vi "raster-scanning_sin_est.vi"() -> ()   [LabVIEW 2017]
uses:
  controls/boolean_info.ctl
  raster-scan-params.ctl
  controls/PI-params.ctl
  fpga_subVIs_ssxy/typeDefs/FXP_ss_control_params_zaxis_sinEst.ctl
  <vilib>/Platform/TimedLoop/XDataNode/timing_clust.ctl
  <vilib>/Platform/TimedLoop/XDataNode/nitl_modes.ctl
  <vilib>/Platform/TimedLoop/XDataNode/wakeup.ctl
  <vilib>/rvi/Emulation/niFpgaGetClockAttributes.vi
  <vilib>/rvi/Emulation/niFpgaSctlEmulationGetInTimedLoop.vi
  <vilib>/rvi/Emulation/niFpgaEmulationReportErrorSimple.vi
  <vilib>/rvi/Emulation/niFpgaCriticalErrorInLSC.vi
  <vilib>/rvi/Memory/Memory_Emulation/nirvimemoryFastEmulation.vi
  <vilib>/rvi/Memory/Memory_Emulation/nirvimemoryEmulation.vi
  <vilib>/rvi/Emulation/niFpgaEmulationIsFPGAContextNoSignature.vi
  <vilib>/rvi/DataTransferAndStorage/Container/Common/niFpgaContainerGetUniqueNameForEmu.vi
  <vilib>/rvi/Emulation/niFpgaProcessEmulError.vi
  <vilib>/rvi/errors/nirviReportUnexpectedCaseInternalError (U32).vi
  <vilib>/rvi/eio/common/nirviEmuTemplateMethod_errors.vi
  <vilib>/rvi/Memory/Memory_Emulation/niFpgaMemoryEmulationCacheClearOnFirstRun.vi
  <vilib>/rvi/Memory/Memory_Emulation/nirvimemoryEmulationManagerCache_MakeExclusive.vi
  <vilib>/rvi/Memory/Memory_Emulation/niFpgaMemoryEmulationValidateCache.vi
  <vilib>/rvi/Memory/Memory_Emulation/nirvimemoryEmulationManagerCache_InsertValue.vi
  <vilib>/Utility/error.llb/Clear Errors.vi
  <vilib>/rvi/Memory/Memory_Emulation/nirvimemoryEmulationManagerCache_ReleaseExclusive.vi
  <vilib>/rvi/Memory/Memory_Emulation/nirvimemoryEmulationManagerCache_GetValue.vi
  <vilib>/rvi/Memory/Memory_Emulation/nirvimemoryEmulationManagerCache_SetValue.vi
  <vilib>/rvi/DataTransferAndStorage/Container/Common/niFpgaContainerExecOnDevCompGetState.vi
  <vilib>/Platform/TimedLoop/XDataNode/XDataNode.xnode
  <vilib>/rvi/DataTransferAndStorage/Container/XNode/niFpgaContainer.xnode
  <vilib>/eio/EIONode/EIONode.xnode
  <vilib>/rvi/DataTransferAndStorage/Register/Emulation/niFpgaRegisterEmulation.vi
  <vilib>/rvi/DataTransferAndStorage/Register/Emulation/niFpgaRegisterEmulationRefIn.vi
  libimaging-cs.lvlib
  FPGA-data-logging.lvlib
  <vilib>/Platform/TimedLoop/XDataNode/XDNodeRunTimeDep.lvlib
panel:
  out "Ns":u8=2
  out "Stopped":bool
  in  "z-axis-ss-control-params":T1={"umax"=3.0, "Ns"=0, "Ns_nsw"=0}
  out "SS FIFO TimeOut?":bool
  out "NS_nsw":u8=2
  in  "raster-scan-params":T2={"TsTicks"=1600, "Stop"=TRUE, "TOL"=0.3, "ramp-rate"=0.0, "z-u-max"=5.0, "PI-params"={"Ki"=0.001, "setpoint"=0.0}, "Num"=[-0.00254, 0.000408, 0.00295, 0.0, 0.0, 0.0, 0.0, 0.0, 0.0], "TF Order"=2, "Den"=[0.982758, -1.98194, 1.0, 0.0, 0.0, 0.0, 0.0, 0.0, 0.0]} {"z-u-max" format="%#_13g"; "TOL" format="%#_13g"}
  in  "Z-settle-N":i16
  in  "do_xy_CL":bool
  in  "do-Dz":bool
  out "boolean errors":T4
  in  "xy-init":fxp<+/-,16,5>[](array[numeric])=[0.0, 0.0]
  in  "Ki-xy":sgl=0.001 format="%#_13g"
  in  "xy-bound":sgl
  in  "trigger-0":bool
  in  "u(0)":sgl format="%#_13g"
  out "e(0) (threshhold init)":fxp<+/-,16,5>
  out "current-case":i16
  out "DAC-zaxis":sgl
  out "ADC-zaxis":fxp<+/-,24,5>
  in  "raise-constant":sgl
  # "DIAGNOSTICS"
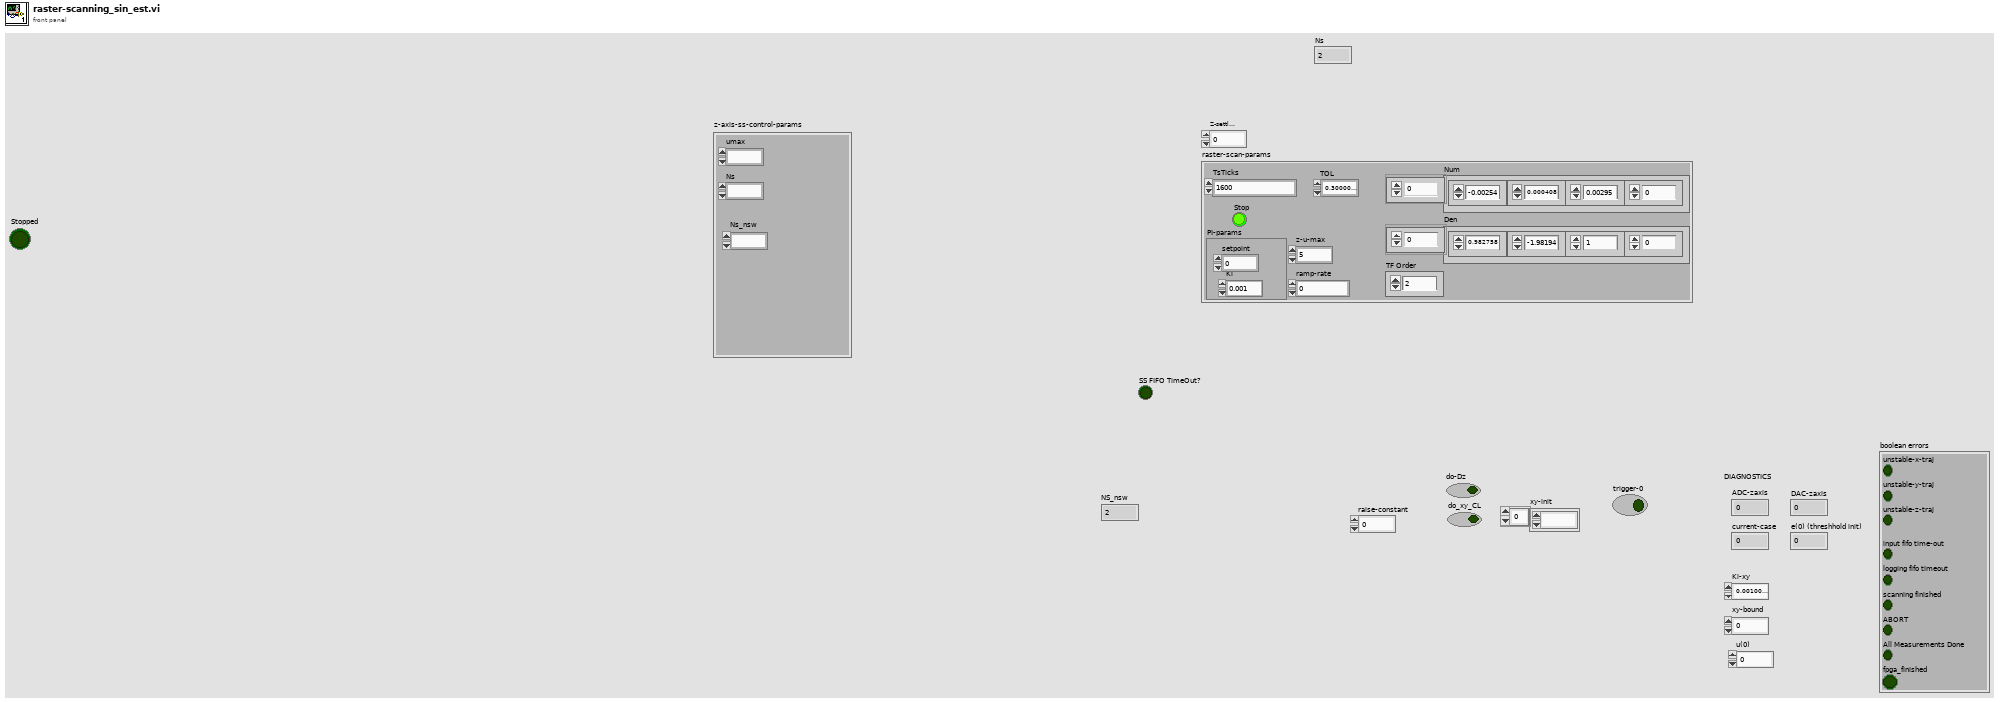
[diagram p1: front panel]
types:
  T1 = typedef "FXP_ss_control_params_zaxis_sinEst.ctl" = cluster{"umax":fxp<+/-,18,5>, "Ns":u8, "Ns_nsw":u8}
  T2 = typedef "raster-scan-params.ctl" = cluster{"TsTicks":u32, "Stop":bool, "TOL":sgl, "ramp-rate":sgl, "z-u-max":sgl, "PI-params":T3, "Num":sgl[], "TF Order":i32, "Den":sgl[]}
  T3 = typedef "PI-params.ctl" = cluster{"Ki":sgl, "setpoint":sgl}
  T4 = typedef "boolean_info.ctl" = cluster{"unstable-z-traj":bool, "input fifo time-out":bool, "logging fifo timeout":bool, "scanning finished":bool, "unstable-x-traj":bool, "unstable-y-traj":bool, "ABORT":bool, "All Measurements Done":bool, "fpga_finished":bool}
  T5 = typedef "XDNodeRunTimeDep.lvlib/timing_clust.ctl" = cluster{"Expected End [f-1]":u64, "Actual End [f-1]":u64, "Finished Late? [f-1]":bool, "Expected End [i-1]":u64, "Actual End [i-1]":u64, "Finished Late? [i-1]":bool, "Expected Start [i]":u64, "Actual Start [i]":u64, "Expected Start [f]":u64, "Actual Start [f]":u64, "Source Name":string, "Structure Name":string, "Period":i64, "Deadline":i64, "Offset":i64, "Start":i64, "Priority":i32, "Timeout":i32, "Mode":T6, "Wakeup Reason":T7, "Error":errorcluster, "Source Type":string, "Secondary Source Type":string, "Global End Time":u64, "Global Start Time":u64, "Frame Duration":u64, "Iteration Duration":u64, "Assigned CPU":i32, "I/O Scan Engine Mode":u32}
  T6 = typedef "XDNodeRunTimeDep.lvlib/nitl_modes.ctl" = enum32{"No Change", "Process missed periods, maintain original phase", "Discard missed periods, maintain original phase", "Process missed periods, ignore original phase", "Discard missed periods, ignore original phase"}
  T7 = typedef "XDNodeRunTimeDep.lvlib/wakeup.ctl" = enum32{"Normal", "Aborted", "Asynchronous wakeup", "Timing source error", "Timed loop error", "Timeout"}
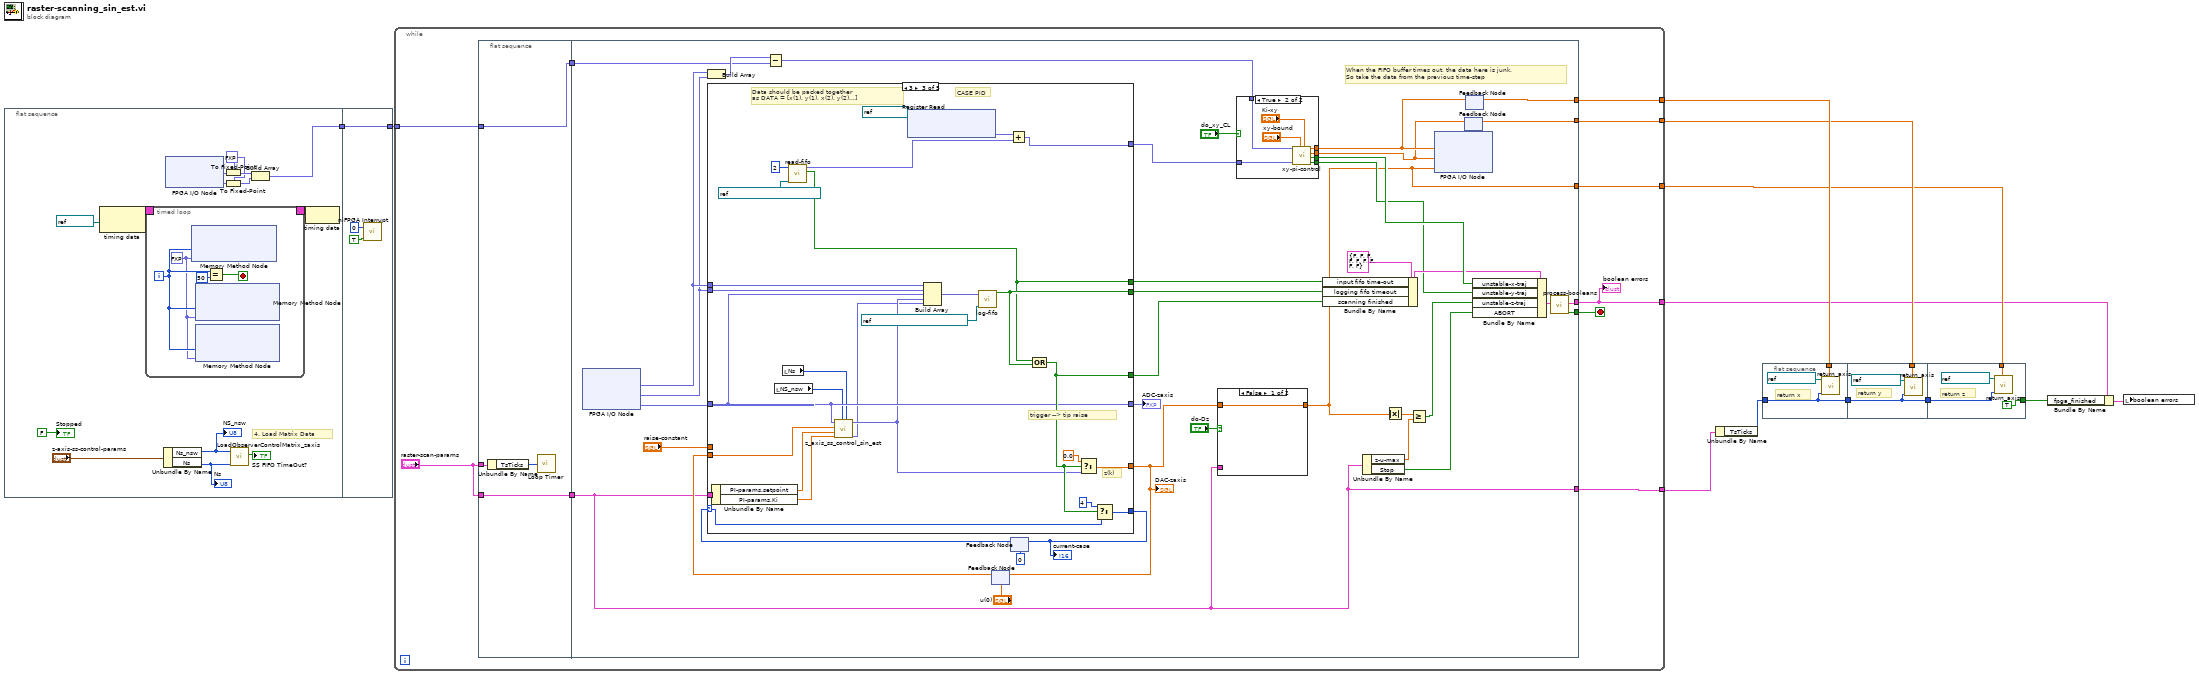
[diagram p0: block diagram]
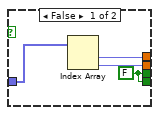
[diagram p2: hidden frame]
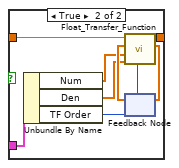
[diagram p3: hidden frame]
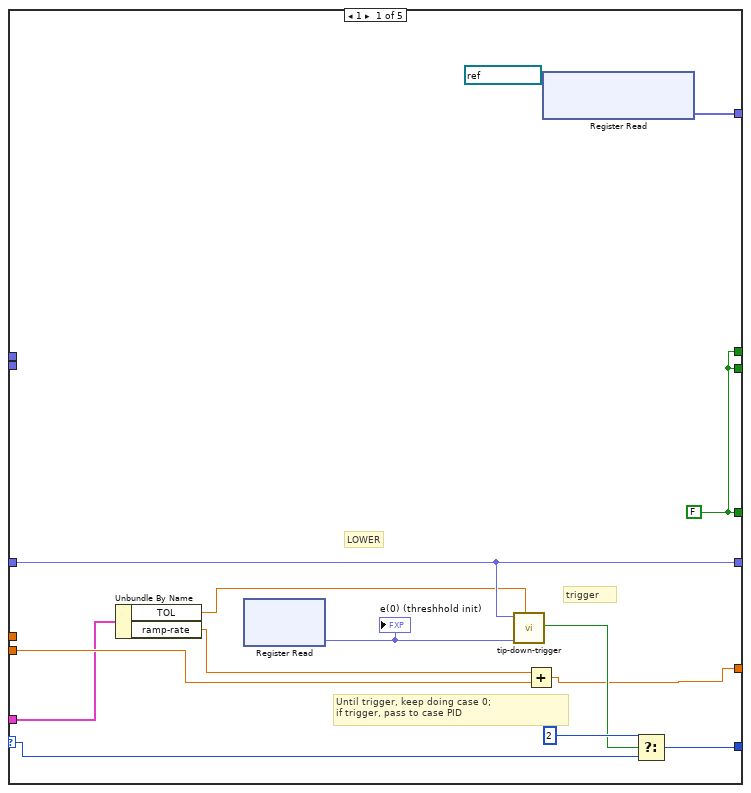
[diagram p4: hidden frame]
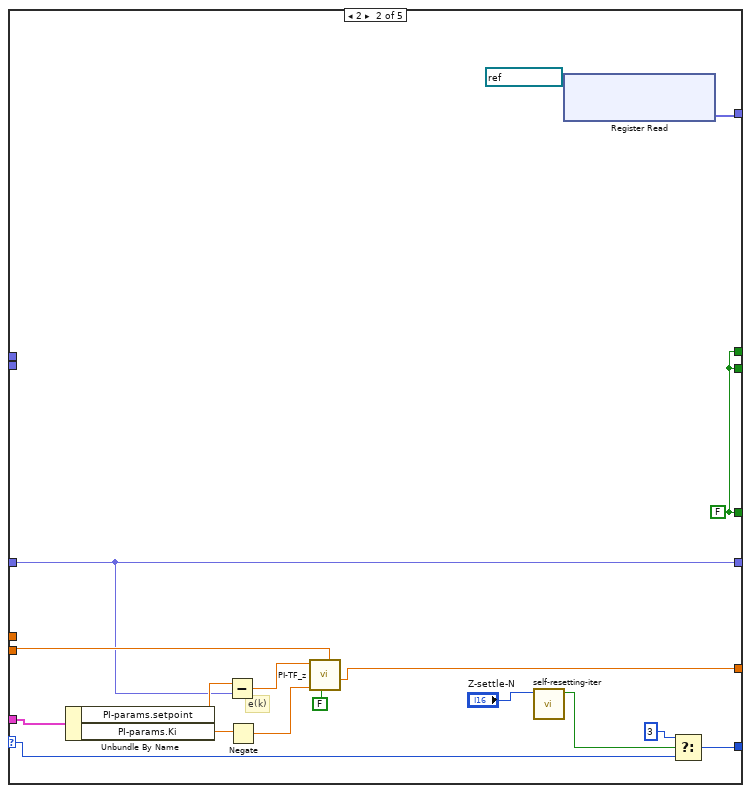
[diagram p5: hidden frame]
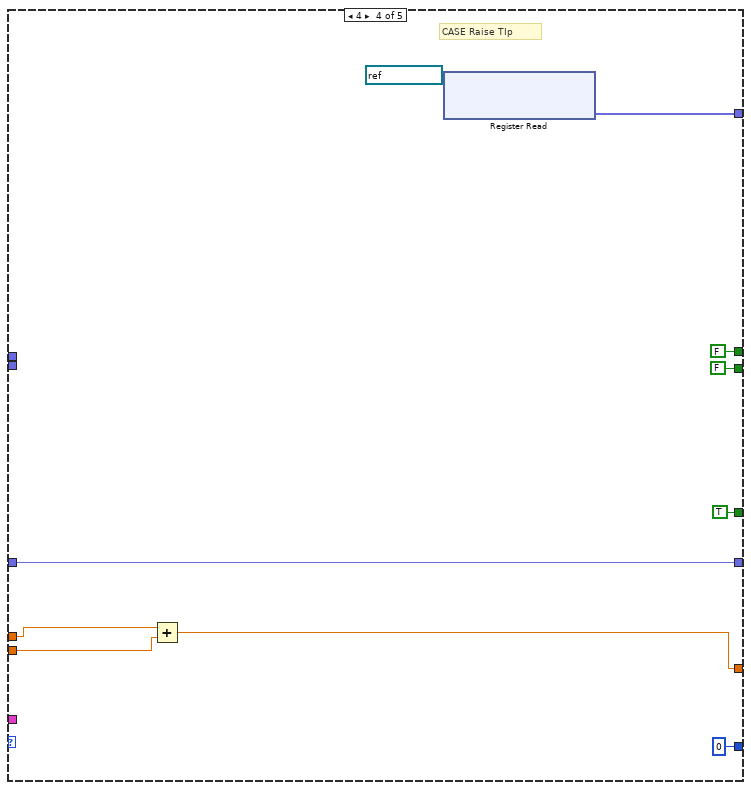
[diagram p6: hidden frame]
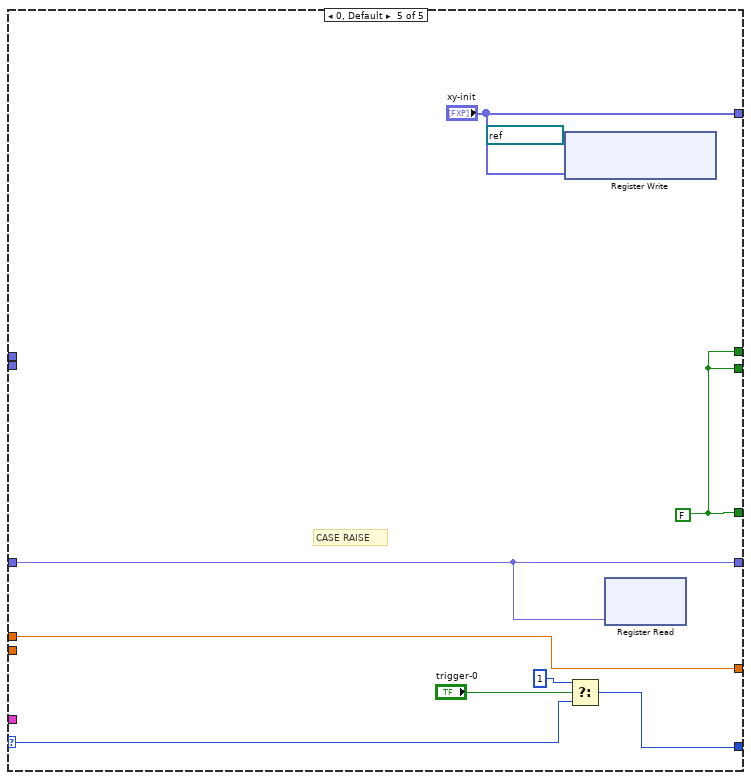
[diagram p7: hidden frame]
diagram:
  n1 = flat-sequence {
    tunnel: [w15] -> w1
    tunnel: [w39] -> w2
    tunnel: w1 -> [w39]
    frame #0 {
      w16 = fxp<+/-,16,5> 0.0 ("fixed-point type")
      # "4. Load Matrix Data"
      n2 = node-c288(refnum<k21> "80MHz" ("Source Name")) -> (w26:T5)
      n3 = timed-loop {
        timing: w26 -> [_]
        timing-out: [_] -> w25
        i -> [w28]
        stop <- w30 stop-if-true
        w27 = fxp<+/-,32,5> 0.0 ("Data")
        n4 = xnode ("Memory Method Node")("Address"=w28, "Data"=w27) -> ()  [unwired: 1 in, 1 out]
        n5 = xnode ("Memory Method Node")("Address"=w28, "Data"=w27) -> ()  [unwired: 1 in, 1 out]
        n6 = xnode ("Memory Method Node")("Address"=w28, "Data"=w27) -> ()  [unwired: 1 in, 1 out]
        n7 = Equal?(x=w28, y=50) -> (x = y?=w30:bool)
      }
      n8 = Unbundle By Name("z-axis-ss-control-params") -> ("Ns_nsw"=w22:u8, "Ns"=w13:u8)
      "NS_nsw" <- w22
      "Ns" <- w13
      n9 = xnode "FPGA I/O Node"() -> ("Mod2/AI0"=w18:fxp<+/-,24,5>, "Mod2/AI1"=w20:fxp<+/-,24,5>)  [unwired: 2 in, 2 out]
      n10 = To Fixed-Point(fixed-point type=w16, number=w18) -> (fixed-point=w17:fxp<+/-,16,5>)
      n11 = To Fixed-Point(fixed-point type=w16, number=w20) -> (fixed-point=w19:fxp<+/-,16,5>)
      n12 = call "LoadObserverControlMatrix_zaxis.vi"("NS"=w13, "NS_nsw"=w22) -> ("SS FIFO TimeOut?"=→"SS FIFO TimeOut?":bool)  [unwired: 9 in]
      n13 = Build Array(w17, w19) -> (w15:fxp<+/-,16,5>[])
      n14 = node-c288(w25) -> ()
      "Stopped" <- FALSE ("Stopped")
    }
    frame #1 {
      n15 = call <vilib>:"niFPGA Interrupt.vi"("Wait Until Cleared (F)"=TRUE, "IRQ Number (0)"=u8 0) -> ()  [unwired: 1 in]
    }
  }
  n16 = while {
    tunnel: [w48] -> w12
    tunnel: [w47] -> w10
    tunnel: [w44] -> w4
    tunnel: [w46] -> w8
    tunnel: [w45] -> w9
    tunnel: w2 -> [w40]
    stop <- w42 stop-if-true
    n17 = flat-sequence {
      tunnel: "raster-scan-params" -> [w52]
      tunnel: [w51] -> w49
      tunnel: "raster-scan-params" -> [w51]
      tunnel: [w50] -> w43
      tunnel: w40 -> [w50]
      tunnel: w49 -> [w60]
      tunnel: [w82] -> w47
      tunnel: [w60] -> w48
      tunnel: [w56] -> w44
      tunnel: [w62] -> w46
      tunnel: [w75] -> w45
      tunnel: w43 -> [w69]
      tunnel: [w54] -> w42
      frame #0 {
        n18 = Unbundle By Name(w52) -> ("TsTicks"=w53:u32)
        n19 = call "Loop Timer"("Count(Ticks)"=w53) -> ()  [unwired: 1 out]
      }
      frame #1 {
        # "When the FIFO buffer times out, the data here is junk.\nSo take the data from the previous time-step"
        n20 = xnode "FPGA I/O Node"() -> ("Mod2/AI0"=w79:fxp<+/-,24,5>, "Mod2/AI1"=w78:fxp<+/-,24,5>, "Mod2/AI2"=w90:fxp<+/-,24,5>)  [unwired: 3 in, 3 out]
        n21 = Build Array(w79, w78) -> (w70:fxp<+/-,24,5>[])
        n22 = Subtract(x=w70, y=w69) -> (x-y=w68:fxp<+/-,25,6>[])
        n23 = feedback #1("u(0)") -> (w85:sgl)
        n24 = feedback #2(i16 0 ("f")) -> (w86:i16)
        n25 = case shown="3" w86 {
          selector: w86 -> [w114 w131 w162 _ w183]
          tunnel: w85 -> [w125 w136 w146 w178 _]
          tunnel: w90 -> [w122 w129 w151 w172 w188]
          tunnel: [w122 w129 w151 w172 w188] -> w89
          tunnel: [w124 w133 w168 i16 0 ("f") w186] -> w87
          tunnel: w78 -> [_ _ w166 _ _]
          tunnel: w79 -> [_ _ w165 _ _]
          tunnel: [w115 w128 w163 TRUE ("Timed Out?") w185] -> w55
          tunnel: [w119 w135 w164 w177 w182] -> w61
          tunnel: w60 -> [w118 w137 w149 _ _]
          tunnel: [w115 w128 w156 FALSE ("Timed Out?") w185] -> w66
          tunnel: [w115 w128 w160 FALSE ("Timed Out?") w185] -> w67
          tunnel: [w112 w126 w153 w170 "xy-init"] -> w74
          tunnel: "raise-constant" -> [_ _ _ w179 w182]
          frame 1 {
            w115 = FALSE ("Timed Out?")
            # "Until trigger, keep doing case 0;\nif trigger, pass to case PID"
            # "LOWER"
            # "trigger"
            n26 = Unbundle By Name(w118) -> ("TOL"=w117:sgl, "ramp-rate"=w116:sgl)
            n27 = xnode ("Register Read")() -> ("Data"=w120:fxp<+/-,16,5>)  [unwired: 1 in, 1 out]
            "e(0) (threshhold init)" <- w120
            n28 = call "tip-down-trigger.vi"("TOL"=w117, "Vo"=w120, "e(k)"=w122) -> ("trigger"=w121:bool)  [unwired: 8 in]
            n29 = Add(x=w116, y=w125) -> (x+y=w119:sgl)
            n30 = xnode ("Register Read")("Register In"=refnum<k21> "xy_init") -> ("Data"=w112:fxp<+/-,17,6>[])  [unwired: 1 out]
            n31 = Select(t=i16 2, s=w121, f=w114) -> (s? t:f=w124:i16)
          }
          frame 2 {
            w128 = FALSE ("Timed Out?")
            # "e(k)"
            n32 = Unbundle By Name(w137) -> ("PI-params.setpoint"=w142:sgl, "PI-params.Ki"=w139:sgl)
            n33 = Subtract(x=w142, y=w129) -> (x-y=w140:sgl)
            n34 = Negate(x=w139) -> (-x=w138:sgl)
            n35 = call "PI-TF_z.vi"("u(k-1)"=w136, "reset"=FALSE, "Ki"=w138, "e(k)"=w140) -> ("u(k)"=w135:sgl)  [unwired: 7 in]
            n36 = call "self-resetting-iter.vi"("N"="Z-settle-N") -> ("Boolean"=w132:bool)  [unwired: 9 in, 1 out]
            n37 = xnode ("Register Read")("Register In"=refnum<k21> "xy_init") -> ("Data"=w126:fxp<+/-,17,6>[])  [unwired: 1 out]
            n38 = Select(t=i16 3, s=w132, f=w131) -> (s? t:f=w133:i16)
          }
          frame 3 {
            # "Data should be packed together\nas DATA = [x(1), y(1), x(2), y(2)...]"
            # "trigger --> tip raise"
            # "z(k)"
            # "CASE PID"
            n39 = Unbundle By Name(w149) -> ("PI-params.setpoint"=w148:sgl, "PI-params.Ki"=w147:sgl)
            n40 = local read "NS_nsw"() -> (w144:u8)
            n41 = local read "Ns"() -> (w143:u8)
            n42 = call "read-fifo.vi"("FIFO In"=refnum<k21> "host-to-fpga-fxp-16-5", "numChan"=2) -> ("timout?"=w156:bool, "unpacked-data"=w152:fxp<+/-,16,5>[])  [unwired: 8 in]
            n43 = call "z_axis_ss_control_sin_est.vi"("NS"=w143, "Ns+Nsd"=w144, "Ki_z"=w147, "r"=w148, "u(k-1)"=w146, "Y(k): x"=w151) -> ("sinusoid_est"=w145:fxp<+/-,32,5>, "u_k (saturated)"=w150:fxp<+/-,32,5>)  [unwired: 4 in]
            n44 = xnode ("Register Read")("Register In"=refnum<k21> "xy_init") -> ("Data"=w154:fxp<+/-,17,6>[])  [unwired: 1 out]
            n45 = Build Array(w165, w166, w151, w150, w145) -> (w161:fxp<+/-,32,5>[])
            n46 = call "log-fifo.vi"("FIFO In"=refnum<k21> "fpga-to-host2-fxp-16-5", "input-data"=w161) -> ("logging-timeout?"=w160:bool)  [unwired: 9 in]
            n47 = Add(x=w154, y=w152) -> (x+y=w153:fxp<+/-,18,7>[])
            n48 = Compound Arithmetic op=OR(w156, w160) -> (w163:bool)
            n49 = Select(t=sgl 0.0 ("f"), s=w163, f=w150) -> (s? t:f=w164:sgl)
            n50 = Select(t=i16 4, s=w163, f=w162) -> (s? t:f=w168:i16)
          }
          frame 4 {
            # "CASE Raise TIp"
            n51 = Add(x=w179, y=w178) -> (x+y=w177:sgl)
            n52 = xnode ("Register Read")("Register In"=refnum<k21> "xy_init") -> ("Data"=w170:fxp<+/-,17,6>[])  [unwired: 1 out]
          }
          frame 0, Default {
            w185 = FALSE ("Timed Out?")
            # "CASE RAISE"
            n53 = xnode ("Register Write")("Data"="xy-init", "Register In"=refnum<k21> "xy_init") -> ()  [unwired: 1 out]
            n54 = Select(t=i16 1 ("f"), s="trigger-0", f=w183) -> (s? t:f=w186:i16)
            n55 = xnode ("Register Read")("Data"=w188) -> ()  [unwired: 1 in, 1 out]
          }
        }
        "ADC-zaxis" <- w89
        "DAC-zaxis" <- w61
        "current-case" <- w87
        n56 = feedback-in #1(w61) -> ()
        n57 = feedback-in #2(w87) -> ()
        n58 = case shown="False" "do-Dz" {
          tunnel: [w103 w109] -> w62
          tunnel: w61 -> [w103 w108]
          tunnel: w60 -> [_ w104]
          frame False {
          }
          frame True {
            n59 = Unbundle By Name(w104) -> ("Num"=w107:sgl[], "Den"=w106:sgl[], "TF Order"=w105:i32)
            n60 = feedback #3() -> (w110:sgl[])  [unwired: 1 in]
            n61 = call "Float_Transfer_Function.vi"("TF Order"=w105, "Den"=w106, "Num"=w107, "State In"=w110, "Input"=w108) -> ("State Out"=w111:sgl[], "Output"=w109:sgl)  [unwired: 4 in]
            n62 = feedback-in #3(w111) -> ()
          }
        }
        n63 = case shown="True" "do_xy_CL" {
          tunnel: [w93 w100] -> w77
          tunnel: [w92 w99] -> w76
          tunnel: w74 -> [w94 w98]
          tunnel: [w91 w97] -> w72
          tunnel: w68 -> [_ w96]
          tunnel: [w91 w95] -> w63
          frame False {
            w91 = FALSE ("u_x saturated")
            n64 = Index Array(array=w94) -> (element #1=w93:fxp<+/-,18,7>, element #2=w92:fxp<+/-,18,7>)  [unwired: 2 in]
          }
          frame True {
            n65 = call "xy-pi-control.vi"("Ki-xy"="Ki-xy", "xy-umax"="xy-bound", "xy-ref"=w98, "x_k-y_k"=w96) -> ("u_y saturated"=w95:bool, "u_x saturated"=w97:bool, "sat(u_y)"=w99:sgl, "sat(u_x)"=w100:sgl)  [unwired: 4 in]
          }
        }
        n66 = Bundle By Name(cluster=T4 {"unstable-z-traj"=FALSE, "input fifo time-out"=FALSE, "logging fifo timeout"=FALSE, "scanning finished"=FALSE, "unstable-x-traj"=FALSE, "unstable-y-traj"=FALSE, "ABORT"=FALSE, "All Measurements Done"=FALSE, "fpga_finished"=FALSE} ("boolean errors 2"), "input fifo time-out"=w66, "logging fifo timeout"=w67, "scanning finished"=w55) -> (w64:T4)
        n67 = Unbundle By Name(w60) -> ("z-u-max"=w83:sgl, "Stop"=w80:bool)
        n68 = Absolute Value(x=w62) -> (abs(x)=w88:sgl)
        n69 = Greater Or Equal?(x=w88, y=w83) -> (x >= y?=w81:bool)
        n70 = xnode "FPGA I/O Node"("Mod1/AO0"=w77, "Mod1/AO1"=w76, "Mod1/AO2"=w62) -> ()  [unwired: 3 in, 3 out]
        n71 = feedback #4() -> (w75:sgl)  [unwired: 1 in]
        n72 = feedback-in #4(w76) -> ()
        n73 = feedback-in #5(w77) -> ()
        n74 = feedback #5() -> (w82:sgl)  [unwired: 1 in]
        n75 = Bundle By Name(cluster=w64, "unstable-x-traj"=w72, "unstable-y-traj"=w63, "unstable-z-traj"=w81, "ABORT"=w80) -> (w57:T4)
        n76 = call "process-booleans.vi"("boolean indicators 2"=w57) -> ("scaning finished"=w54:bool, "boolean indicators"=w56:T4)  [unwired: 9 in]
      }
    }
    "boolean errors" <- w44
  }
  n77 = Unbundle By Name(w12) -> ("TsTicks"=w11:u32)
  n78 = flat-sequence {
    tunnel: w11 -> [w190]
    tunnel: w10 -> [w191]
    tunnel: [w190] -> w7
    tunnel: w9 -> [w194]
    tunnel: w7 -> [w192]
    tunnel: [w192] -> w6
    tunnel: w8 -> [w198]
    tunnel: w6 -> [w196]
    tunnel: [TRUE] -> w5
    frame #0 {
      # "return x"
      n79 = call "return_axis.vi"("u(0)"=w191, "TsTicks"=w190, "FPGA I/O In"=refnum<k21> "Mod1/AO0") -> ()  [unwired: 9 in]
    }
    frame #1 {
      # "return y"
      n80 = call "return_axis.vi"("u(0)"=w194, "TsTicks"=w192, "FPGA I/O In"=refnum<k21> "Mod1/AO1") -> ()  [unwired: 9 in]
    }
    frame #2 {
      # "return z"
      n81 = call "return_axis.vi"("u(0)"=w198, "TsTicks"=w196, "FPGA I/O In"=refnum<k21> "Mod1/AO2") -> ()  [unwired: 9 in]
    }
  }
  n82 = Bundle By Name(cluster=w4, "fpga_finished"=w5) -> (w3:T4)
  n83 = local write "boolean errors"(w3) -> ()
